vi "Slide Splitter.vi"(4 "Message XML":refnum<vi>, 6 "Hidden Pane":refnum<vi>, 7 "Splitter":refnum<vi>, 9 "New Value":i32, 10 "Old Value":i32) -> ()   [LabVIEW 2017, in "MGI-Monitored Actor.lvlib" / "Classic Logger.lvclass"]
uses:
  Classic Logger.lvclass
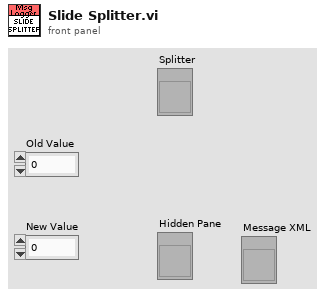
[diagram p1: front panel]
types:
  T1 = enum16{"No Scaling", "Scale All Objects", "Scale Single Object"}
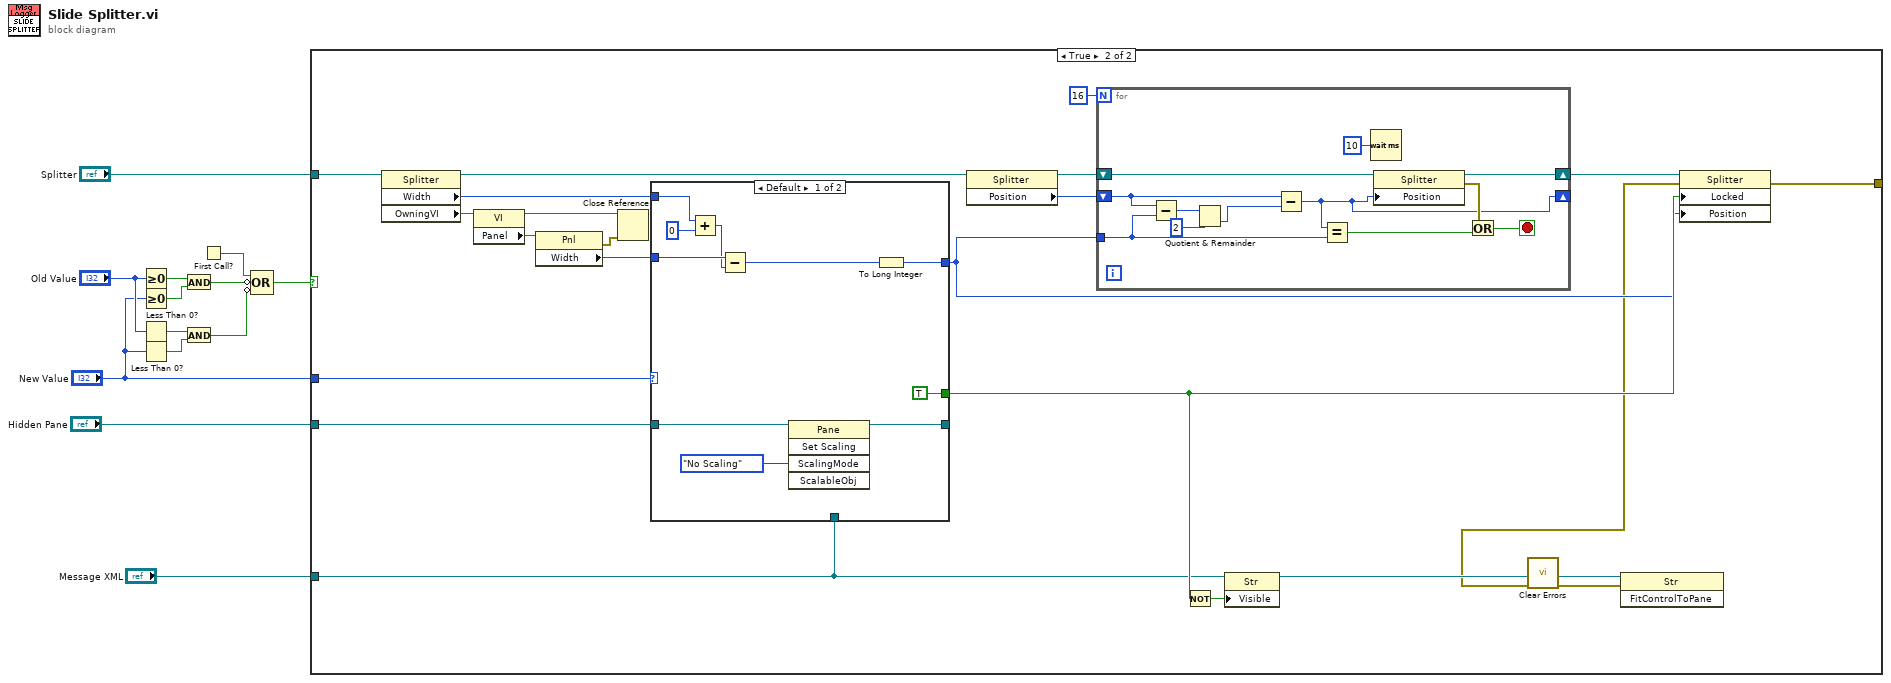
[diagram p0: block diagram]
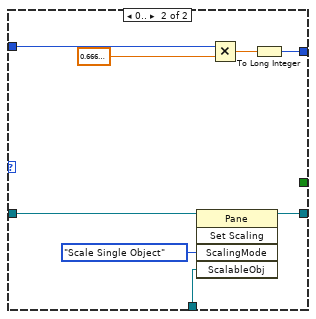
[diagram p3: hidden frame]
diagram:
  n1 = Greater Or Equal To 0?(x="Old Value") -> (x >= 0?=w12:bool)
  n2 = Greater Or Equal To 0?(x="New Value") -> (x >= 0?=w11:bool)
  n3 = Less Than 0?(x="Old Value") -> (x < 0?=w9:bool)
  n4 = Less Than 0?(x="New Value") -> (x < 0?=w10:bool)
  n5 = And(x=w12, y=w11) -> (x .and. y?=w7:bool)
  n6 = And(x=w9, y=w10) -> (x .and. y?=w6:bool)
  n7 = First Call?() -> (First Call?: T/F=w1:bool)
  n8 = Compound Arithmetic op=OR(w1, invert w7, invert w6) -> (w5:bool)
  n9 = case shown="True" w5 {
    tunnel: "Splitter" -> [_ w32]
    tunnel: "New Value" -> [_ w24]
    tunnel: [_ w15] -> _
    tunnel: "Hidden Pane" -> [_ w22]
    tunnel: "Message XML" -> [_ w17]
    frame False {
      # "Already in the correct position"
    }
    frame True {
      n10 = property class="Splitter"(reference=w32) -> (reference out=w26:refnum<vi>, "Width"=w25:u32, "OwningVI"=w31:refnum<vi>)  [unwired: 1 in, 1 out]
      n11 = property class="VI"(reference=w31) -> (reference out=w29:refnum<vi>, "Panel"=w30:refnum<vi>)  [unwired: 1 in, 1 out]
      n12 = property class="Pnl"(reference=w30) -> (error out=w27:errorcluster, "Width"=w28:u32)  [unwired: 1 in, 1 out]
      n13 = Close Reference(reference=w29, error in (no error)=w27) -> ()  [unwired: 1 out]
      n14 = case shown="Default" w24 {
        tunnel: w28 -> [w44 w52]
        tunnel: [w41 w49] -> w20
        tunnel: w25 -> [w40 _]
        tunnel: [TRUE _] -> w23
        tunnel: w22 -> [w36 w48]
        tunnel: w17 -> [_ w46]
        tunnel: [w35 w45] -> _
        frame Default {
          n15 = Add(x=w40, y=u32 0) -> (x+y=w38:u32)
          n16 = Subtract(x=w44, y=w38) -> (x-y=w43:u32)
          n17 = invoke class="Pane" method="Set Scaling"(reference=w36, "ScalingMode"=T1."No Scaling" ("Scaling Mode")) -> (reference out=w35:refnum<vi>)  [unwired: 3 in, 4 out]
          n18 = To Long Integer(number=w43) -> (32bit integer=w41:i32)
        }
        frame 0.. {
          n19 = invoke class="Pane" method="Set Scaling"(reference=w48, "ScalingMode"=T1."Scale Single Object" ("Scaling Mode"), "ScalableObj"=w46) -> (reference out=w45:refnum<vi>)  [unwired: 2 in, 4 out]
          n20 = Multiply(x=w52, y=sgl 0.666) -> (x*y=w50:sgl)
          n21 = To Long Integer(number=w50) -> (32bit integer=w49:i32)
        }
      }
      n22 = property class="Splitter"(reference=w26) -> (reference out=w34:refnum<vi>, "Position"=w21:i32)  [unwired: 1 in, 1 out]
      n23 = for {
        N: 16 -> [_]
        shift-right: [w63] -> w33
        shift-left: w34 -> [w64]
        shift-right: [w59] -> _
        shift-left: w21 -> [w57]
        tunnel: w20 -> [w56]
        stop <- w58 stop-if-true
        n24 = Subtract(x=w57, y=w56) -> (x-y=w55:i32)
        n25 = Quotient & Remainder(x=w55, y=2) -> (floor(x/y)=w53:i32)  [unwired: 1 out]
        n26 = Subtract(x=w57, y=w53) -> (x-y=w59:i32)
        n27 = Equal?(x=w59, y=w56) -> (x = y?=w60:bool)
        n28 = Wait (ms)(milliseconds to wait=u32 10) -> ()  [unwired: 1 out]
        n29 = property class="Splitter"(reference=w64, "Position"=w59) -> (reference out=w63:refnum<vi>, error out=w61:errorcluster)  [unwired: 1 in]
        n30 = Or(x=w61, y=w60) -> (x .or. y?=w58:bool)
      }
      n31 = Not(x=w23) -> (.not. x?=w18:bool)
      n32 = property class="Str"(reference=w17, "Visible"=w18) -> (reference out=w16:refnum<vi>)  [unwired: 1 in, 1 out]
      n33 = property class="Splitter"(reference=w33, "Locked"=w23, "Position"=w20) -> (error out=w15:errorcluster)  [unwired: 1 in, 1 out]
      n34 = call <vilib>:"Clear Errors.vi"("error in (no error)"=w15) -> ("error out"=w14:errorcluster)  [unwired: 5 in, 1 out]
      n35 = invoke class="Str" method="FitControlToPane"(reference=w16, error in=w14) -> ()  [unwired: 1 in, 3 out]
    }
  }
